vi "destroy.vi"(0 "HGF_Reference":refnum<class "HGF_Reference.lvclass">, 2 "wait for activity? (F)":bool, 3 "timeout /ms (-1)":i32=-1, 5 "error in (no error)":errorcluster) -> (14 "Object":refnum<class>, 19 "error out":errorcluster)   [LabVIEW 2014, in "HGF_BaseClasses.lvlib" / "HGF_Reference.lvclass"]
doc: "Destroys the Reference object and returns the referenced object."
uses:
  HGF_Reference.lvclass
  HGF_Reference.lvclass/HGF_Reference.ctl
panel:
  out "timed out?":bool
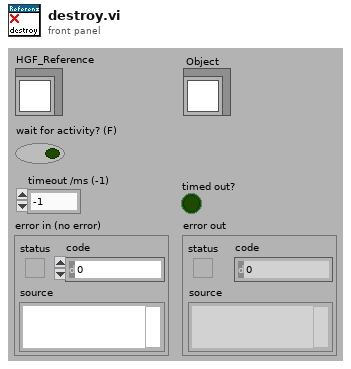
[diagram p1: front panel]
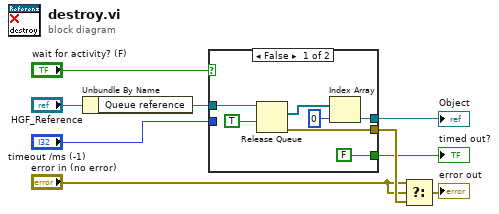
[diagram p0: block diagram]
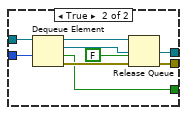
[diagram p2: hidden frame]
diagram:
  n1 = Unbundle By Name("HGF_Reference") -> ("Queue reference"=w9:refnum<queue>)
  n2 = case shown="False" "wait for activity? (F)" {
    tunnel: w9 -> [w14 w24]
    tunnel: [w16 w21] -> w8
    tunnel: [w13 w20] -> w2
    tunnel: "timeout /ms (-1)" -> [_ w19]
    tunnel: [FALSE ("timed out?") w18] -> w1
    frame False {
      n3 = Release Queue(queue=w14, force destroy? (F)=TRUE ("force destroy?")) -> (remaining elements=w15:refnum<class>[], error out=w16:errorcluster)  [unwired: 1 in, 1 out]
      n4 = Index Array(array=w15, index=0) -> (element=w13:refnum<class>)
    }
    frame True {
      n5 = Dequeue Element(queue=w24, timeout in ms (-1)=w19) -> (queue out=w22:refnum<queue>, element=w20:refnum<class>, timed out?=w18:bool, error out=w23:errorcluster)  [unwired: 1 in]
      n6 = Release Queue(queue=w22, force destroy? (F)=FALSE, error in (no error)=w23) -> (error out=w21:errorcluster)  [unwired: 2 out]
    }
  }
  "Object" <- w2
  "timed out?" <- w1
  n7 = Select(t="error in (no error)", s="error in (no error)", f=w8) -> (s? t:f=→"error out":errorcluster)
